vi "blowfish_decipher.vi"(8 "error in (no error)":errorcluster, 11 "Input Text":string) -> (0 "error out":errorcluster, 3 "data string":string)   [LabVIEW 2020]
doc: "The Blowfish Encryption Algorithm\n\nBlock cipher: 64-bit block \nVariable key length: 32 bits to 448 bits \nDesigned by Bruce Schneier \nMuch faster than DES and IDEA \nUnpatented and royalty-free \nNo license required \n\nBlowfish is a symmetric block cipher that can be used as a drop-in replacement for DES or IDEA. It takes a variable-length key, from 32 bits to 448 bits, making it ideal for both domestic and exportable use. Blowfish was designed in 1993 by Bruce Schneier as a fast, free alternative to existing encryption algorithms. Since then it has been analyzed considerably, and it is slowly gaining acceptance as a strong encryption algorithm. Blowfish is unpatented and license-free, and is available free for all uses.\n\nAs far as I know this is the first implementation of the Blowfish Algorithm in LabVIEW. With this set of subvi's one can encrypt data in LabVIEW without the need of external software. This can be used to send data securely over Data socket as well as TCP and UDP communications. And also protect remote control systems from unauthorized access, by encrypting the control communications.\n\nI welcome any constructive commits, and bug reports can be sent to the E-mail contained in the code"
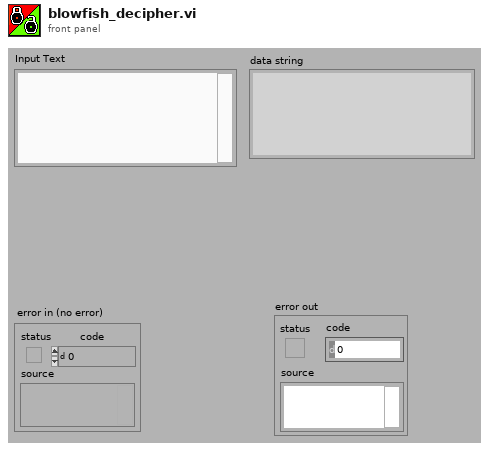
[diagram p1: front panel]
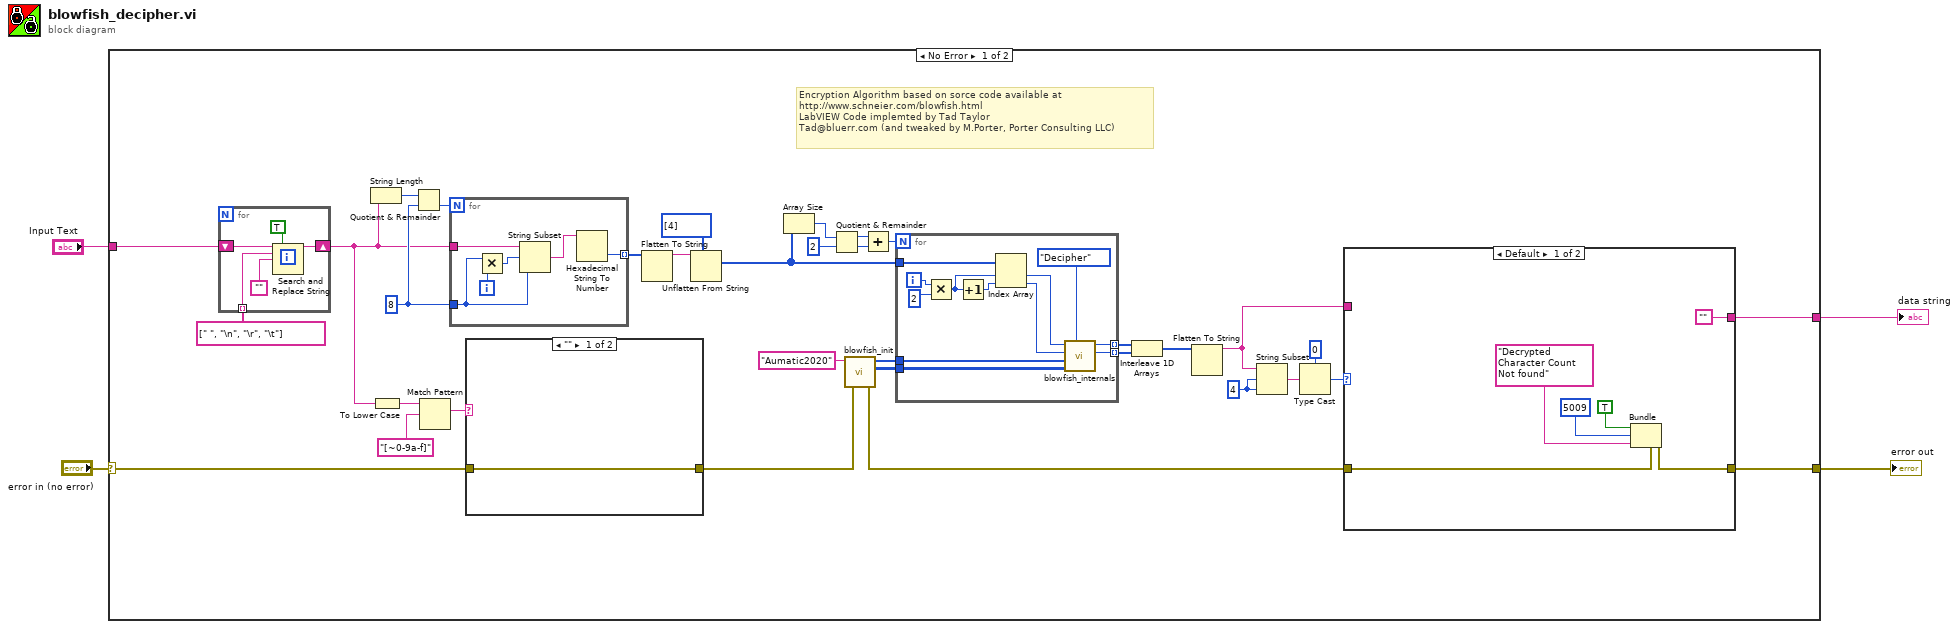
[diagram p0: block diagram]
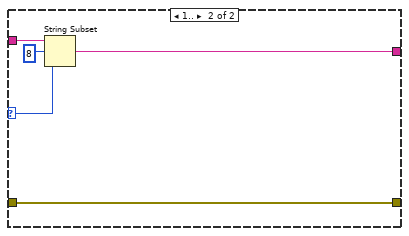
[diagram p2: hidden frame]
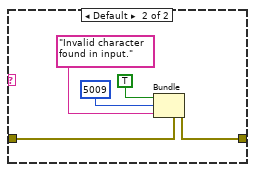
[diagram p3: hidden frame]
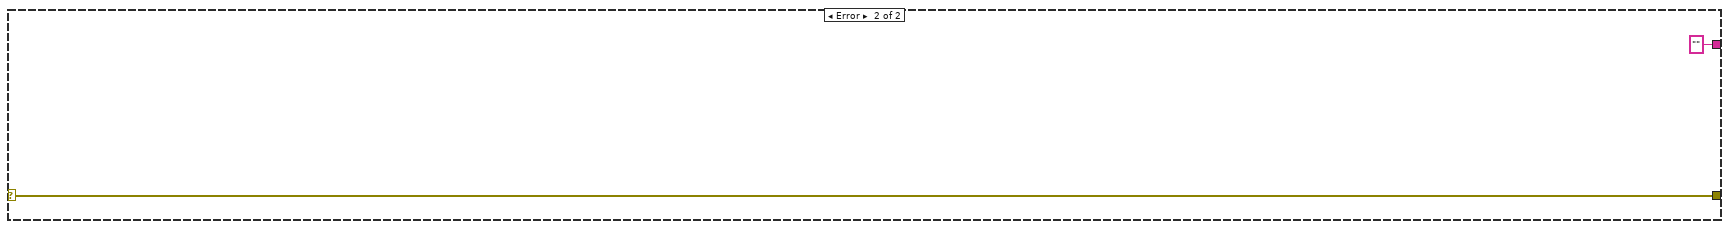
[diagram p4: hidden frame]
diagram:
  n1 = case shown="No Error" "error in (no error)" {
    selector: "error in (no error)" -> [w30 w79]
    tunnel: [w24 "" ("data string")] -> w1
    tunnel: [w23 w79] -> w3
    tunnel: "Input Text" -> [w5 _]
    frame No Error {
      w10 = 4 ("offset (0)")
      w20 = 8 ("length (rest)")
      # "Encryption Algorithm based on sorce code available at\nhttp://www.schneier.com/blowfish.html\nLabVIEW Code implemted by Tad Taylor\nTad@bluerr.com (and tweaked by M.Porter, Porter Consulting LLC)"
      n2 = for {
        shift-right: [w59] -> w14
        shift-left: w5 -> [w60]
        tunnel: string[] [" ", "\n", "\r", "\t"] -> [w57] mode=indexing
        n3 = Search and Replace String(replace all?=TRUE ("replace all? (F)"), input string=w60, search string=w57, replace string="") -> (result string=w59:string)  [unwired: 4 in, 3 out]
      }
      n4 = String Length(string=w14) -> (length=w17:i32)
      n5 = To Lower Case(string=w14) -> (all lower case string=w12:string)
      n6 = Quotient & Remainder(x=w17, y=w20) -> (floor(x/y)=w19:i32)  [unwired: 1 out]
      n7 = Match Pattern(string=w12, regular expression="[~0-9a-f]") -> (match substring=w11:string)  [unwired: 1 in, 3 out]
      n8 = for {
        N: w19 -> [_]
        tunnel: w14 -> [w65]
        tunnel: [w66] -> w21 mode=indexing
        tunnel: w20 -> [w61]
        i -> [w63]
        n9 = Multiply(x=w61, y=w63) -> (x*y=w62:i32)
        n10 = String Subset(string=w65, offset (0)=w62, length (rest)=w61) -> (substring=w64:string)
        n11 = Hexadecimal String To Number(string=w64) -> (number=w66:u32)  [unwired: 2 in, 1 out]
      }
      n12 = case shown="\"\"" w11 {
        tunnel: w30 -> [w50 w55]
        tunnel: [w50 w54] -> w31
        frame "" {
        }
        frame Default {
          n13 = Bundle(cluster=w55, "status"=TRUE ("Halt?"), "code"=5009 ("Halt Code"), "source"="Invalid character found in input." ("Halt Message")) -> (w54:errorcluster)
        }
      }
      n14 = Flatten To String(anything=w21) -> (data string=w16:string)  [unwired: 3 in, 2 out]
      n15 = Unflatten From String(type=u32[] [4] ("appended array"), binary string=w16) -> (value=w33:u32[])  [unwired: 3 in, 2 out]
      n16 = Array Size(array=w33) -> (size(s)=w29:i32)
      n17 = Quotient & Remainder(x=w29, y=2 ("x")) -> (x-y*floor(x/y)=w25:i32, floor(x/y)=w26:i32)
      n18 = call "blowfish_init.vi"("error in (no error)"=w31, "Key"="Aumatic2020") -> ("error out"=w32:errorcluster, "S 4X256"=w37:u32[][], "P 18"=w38:u32[])  [unwired: 3 in]
      n19 = Add(x=w25, y=w26) -> (x+y=w27:i32)
      n20 = for {
        N: w27 -> [_]
        tunnel: [w70] -> w36 mode=indexing
        tunnel: [w69] -> w35 mode=indexing
        tunnel: w38 -> [w73]
        tunnel: w37 -> [w74]
        tunnel: w33 -> [w78]
        i -> [w77]
        n21 = Multiply(x=w77, y=2 ("element")) -> (x*y=w76:i32)
        n22 = Increment(x=w76) -> (x+1=w68:i32)
        n23 = Index Array(array=w78, index #1=w76, index #2=w68) -> (element #1=w72:u32, element #2=w71:u32)
        n24 = call "blowfish_internals.vi"("Enc/Dec"=enum16{"Encipher", "Decipher"}."Decipher", "S 4X256"=w74, "P 18"=w73, "Xr"=w71, "Xl"=w72) -> ("Xr out"=w69:u32, "Xl out"=w70:u32)  [unwired: 2 in]
      }
      n25 = Interleave 1D Arrays(w36, w35) -> (w34:u32[])
      n26 = Flatten To String(anything=w34) -> (data string=w6:string)  [unwired: 3 in, 2 out]
      n27 = String Subset(string=w6, offset (0)=w10, length (rest)=w10) -> (substring=w9:string)
      n28 = Type Cast(type=0 ("offset (0)"), x=w9) -> (*(type *) &x=w7:i32)
      n29 = case shown="Default" w7 {
        selector: w7 -> [_ w48]
        tunnel: w6 -> [_ w49]
        tunnel: ["" ("data string") w45] -> w24
        tunnel: w32 -> [w43 w46]
        tunnel: [w42 w46] -> w23
        frame Default {
          n30 = Bundle(cluster=w43, "status"=TRUE ("Halt?"), "code"=5009 ("Halt Code"), "source"="Decrypted Character Count Not found" ("Halt Message")) -> (w42:errorcluster)
        }
        frame 1.. {
          n31 = String Subset(string=w49, offset (0)=8, length (rest)=w48) -> (substring=w45:string)
        }
      }
    }
    frame Error {
    }
  }
  "error out" <- w3
  "data string" <- w1
